vi "Configure Trigger.vi"(8 "error in (no error)":errorcluster, 9 "Hardware Trigger Delay (0 s)":u16, 10 "Trigger Type (0:Normal)":u8(ring) items=["Normal", "Software Trigger Mode", "External Sync Trigger Mode", "External Hardware Trigger Mode"], 11 "VISA resource name":refnum<visa-resource-name>) -> (0 "error out":errorcluster, 3 "VISA resource name out":refnum<visa-resource-name>)   [LabVIEW 2018, in "Ocean Optics 2000 4000.lvlib"]
doc: "Configures the instrument triggering mode and the Hardware Trigger Delay."
uses:
  Ocean Optics 2000 4000.lvlib
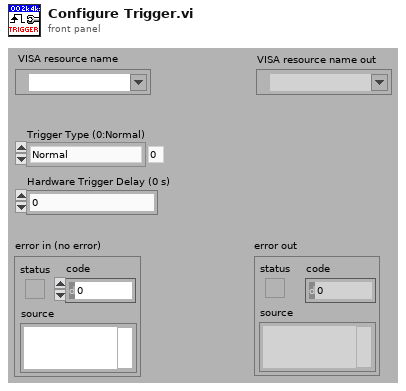
[diagram p1: front panel]
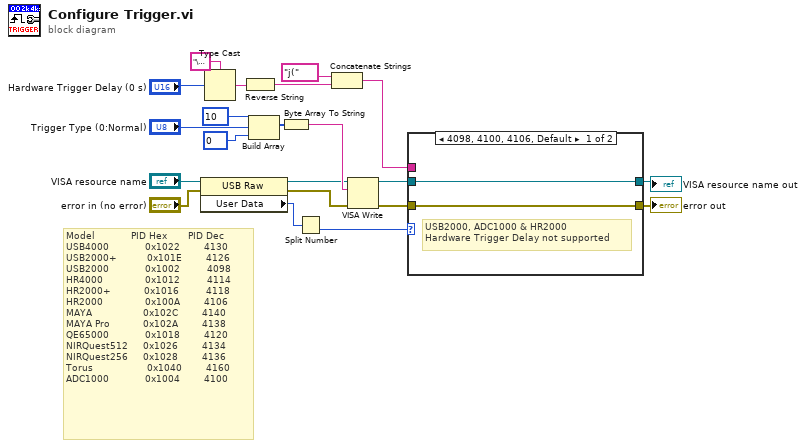
[diagram p0: block diagram]
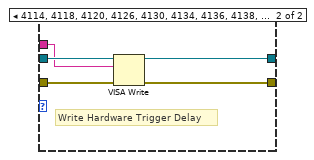
[diagram p2: hidden frame]
diagram:
  # "Model            PID Hex       PID Dec \nUSB4000            0x1022        4130 \nUSB2000+          0x101E        4126 \nUSB2000            0x1002         4098\nHR4000              0x1012         4114\nHR2000+           0x1016         4118\nHR2000              0x100A        4106\nMAYA                 0x102C        4140\nMAYA Pro           0x102A        4138\nQE65000            0x1018        4120\nNIRQuest512     0x1026        4134\nNIRQuest256     0x1028        4136\nTorus                  0x1040        4160\nADC1000            0x1004        4100"
  n1 = property class="USB Raw"(reference="VISA resource name", error in="error in (no error)") -> (reference out=w6:refnum<visa-resource-name>, error out=w5:errorcluster, "User Data"=w2:u32)
  n2 = Type Cast(type="\u0000", x="Hardware Trigger Delay (0 s)") -> (*(type *) &x=w9:string)
  n3 = Reverse String(1:w9) -> (0:w8:string)
  n4 = Build Array(u8 10, "Trigger Type (0:Normal)", u8 0) -> (w20:u8[])
  n5 = Byte Array To String(unsigned byte array=w20) -> (string=w19:string)
  n6 = Split Number(x=w2) -> (lo(x)=w1:u16)  [unwired: 1 out]
  n7 = Concatenate Strings("j(" ("string"), w8) -> (w7:string)
  n8 = VISA Write(VISA resource name=w6, write buffer=w19, error in (no error)=w5) -> (VISA resource name out=w14:refnum<visa-resource-name>, error out=w13:errorcluster)  [unwired: 1 out]
  n9 = case shown="4098, 4100, 4106, Default" w1 {
    tunnel: [w23 w28] -> w16
    tunnel: [w22 w27] -> w15
    tunnel: w14 -> [w23 w26]
    tunnel: w13 -> [w22 w25]
    tunnel: w7 -> [_ w24]
    frame 4098, 4100, 4106, Default {
      # "USB2000, ADC1000 & HR2000\nHardware Trigger Delay not supported"
    }
    frame 4114, 4118, 4120, 4126, 4130, 4134, 4136, 4138, 4140, 4160 {
      # "Write Hardware Trigger Delay"
      n10 = VISA Write(VISA resource name=w26, write buffer=w24, error in (no error)=w25) -> (VISA resource name out=w28:refnum<visa-resource-name>, error out=w27:errorcluster)  [unwired: 1 out]
    }
  }
  "VISA resource name out" <- w16
  "error out" <- w15
